vi "_USB_CAN_BI_.vi"(11 "BOARD_INFO":T1) -> (2 "change?":bool, 3 "BOARD_INFO out":T1)   [LabVIEW 2011]
panel:
  in  "new_SN":string caption="新设备序号："
  in  "ok":bool
  out "str_USB_Serial":string caption="当前设备序号："
  out "str_hw_Type":string caption="硬件类型："
  out "str_Serial_Num":string caption="板卡序列号："
  out "reserved":u8 caption="保留："
  out "can_Num":u8 caption="can通道数："
  out "irq_Num":u16 caption="保留："
  out "in_Ver":string caption="驱动库版本："
  out "dr_Ver":string caption="驱动版本："
  out "fw_Ver":string caption="软件版本："
  out "hw_Ver":string caption="硬件版本："
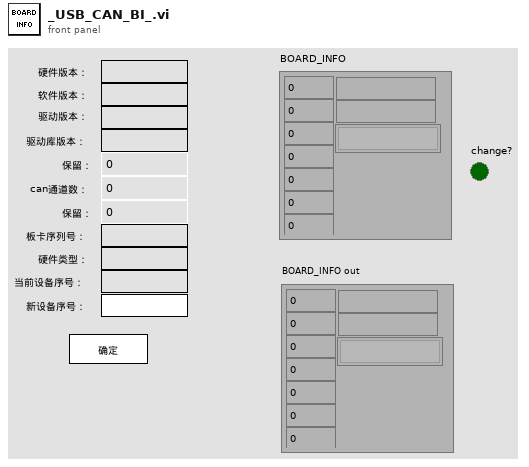
[diagram p1: front panel]
types:
  T1 = cluster{"hw_Version":u16, "fw_Version":u16, "dr_Version":u16, "in_Version":u16, "irq_Num":u16, "can_Num":u8, "reserved":u8, "str_Serial_Num":string, "str_hw_Type":string, "str_GYUsb_Serial":string[]}
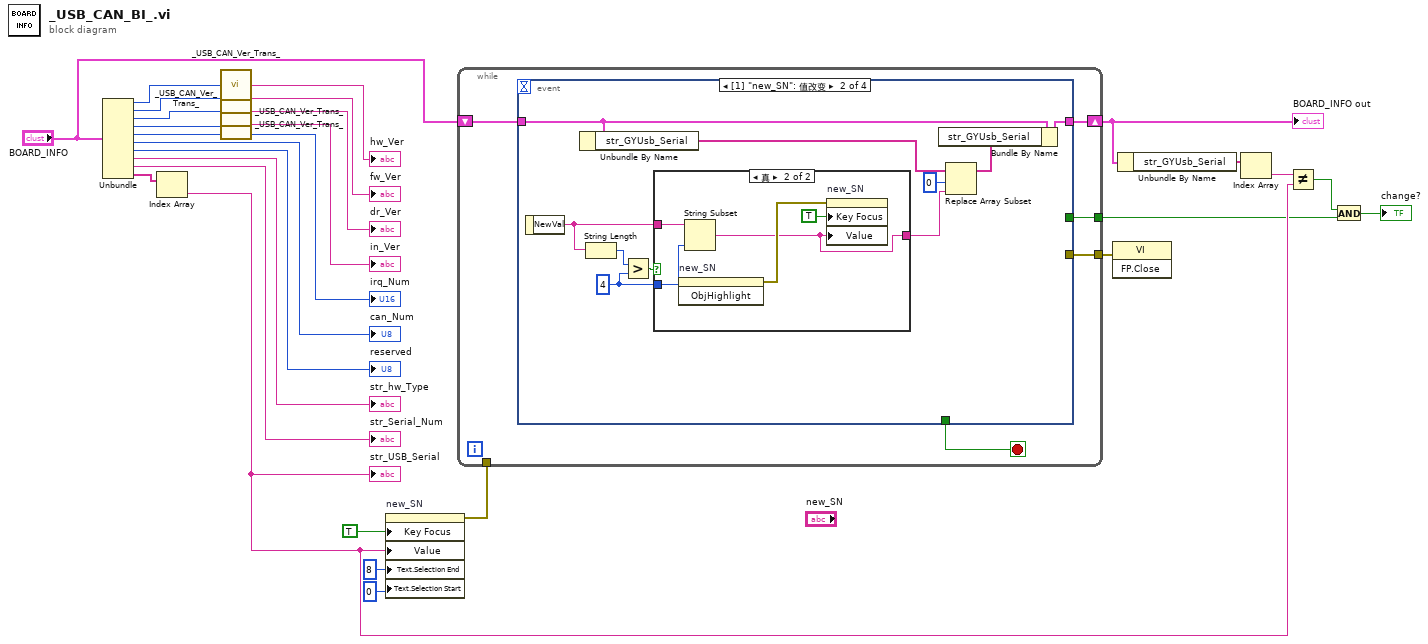
[diagram p0: block diagram]
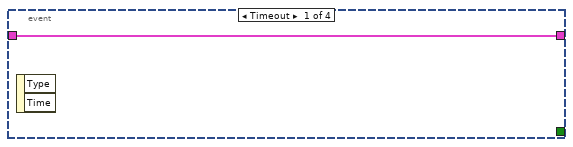
[diagram p2: hidden frame]
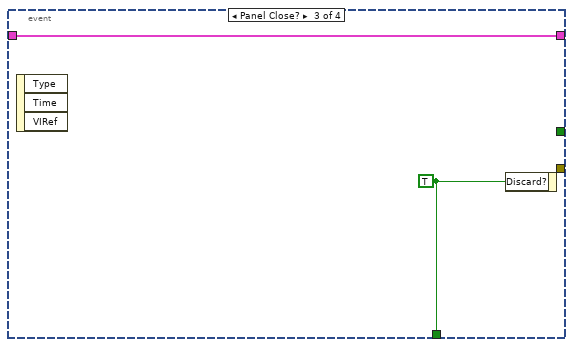
[diagram p4: hidden frame]
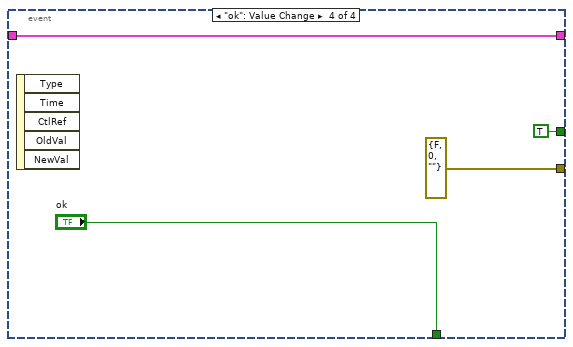
[diagram p5: hidden frame]
diagram:
  n1 = Unbundle("BOARD_INFO") -> ("hw_Version"=w20:u16, "fw_Version"=w19:u16, "dr_Version"=w18:u16, "in_Version"=w17:u16, "irq_Num"=→"irq_Num":u16, "can_Num"=→"can_Num":u8, "reserved"=→"reserved":u8, "str_Serial_Num"=→"str_hw_Type":string, "str_hw_Type"=→"str_Serial_Num":string, "str_GYUsb_Serial"=w22:string[])
  n2 = Index Array(array=w22) -> (element=w6:string)  [unwired: 1 in]
  "str_USB_Serial" <- w6
  n3 = call "_USB_CAN_Ver_Trans_.vi"("u16Ver"=w20) -> ("strVer"=→"hw_Ver":string)
  n4 = call "_USB_CAN_Ver_Trans_.vi"("u16Ver"=w19) -> ("strVer"=→"fw_Ver":string)
  n5 = call "_USB_CAN_Ver_Trans_.vi"("u16Ver"=w18) -> ("strVer"=→"dr_Ver":string)
  n6 = call "_USB_CAN_Ver_Trans_.vi"("u16Ver"=w17) -> ("strVer"=→"in_Ver":string)
  n7 = property on="new_SN" class="Str"("Key Focus"=TRUE ("键选中"), "Value"=w6, "Text.Selection End"=u32 8 ("文本.选择区域:末尾"), "Text.Selection Start"=u32 0 ("文本.选择区域:起始")) -> (error out=w11:errorcluster)  [unwired: 2 in, 1 out]
  n8 = while {
    tunnel: [w31] -> w21
    tunnel: w11 -> [_]
    shift-right: [w30] -> w9
    shift-left: "BOARD_INFO" -> [w29]
    tunnel: [w28] -> w5
    stop <- w32 stop-if-true
    n9 = event shown="[1] \"new_SN\": 值改变" {
      selector: _ -> [_ _ _ _]
      dyn-events: _ -> [_ _ _ _]
      timeout: _ -> [_ _ _ _]
      tunnel: [_ _ w51 "ok"] -> w32
      tunnel: [_ _ _ errorcluster {"status"=FALSE, "code"=0, "source"=""} ("错误输入（无错误）")] -> w31
      tunnel: [w33 w39 w50 w53] -> w30
      tunnel: w29 -> [w33 w38 w50 w53]
      tunnel: [_ _ _ TRUE ("放弃？")] -> w28
      event Timeout {
        n10 = event-data() -> ()  [unwired: 1 in, 2 out]
      }
      event "new_SN": Value Change {
        w40 = 4 ("y")
        n11 = event-data() -> ("NewVal"=w41:string)  [unwired: 1 in]
        n12 = Unbundle By Name(w38) -> ("str_GYUsb_Serial"=w37:string[])
        n13 = String Length(string=w41) -> (length=w43:i32)
        n14 = Greater?(x=w43, y=w40) -> (0:w42:bool)
        n15 = case shown="真" w42 {
          tunnel: w41 -> [w44 w49]
          tunnel: w40 -> [_ w48]
          tunnel: [w44 w45] -> w35
          frame False {
          }
          frame True {
            n16 = invoke on="new_SN" class="Str" method="ObjHighlight"() -> (error out=w46:errorcluster)  [unwired: 3 in, 2 out]
            n17 = String Subset(string=w49, length (rest)=w48) -> (substring=w45:string)  [unwired: 1 in]
            n18 = property on="new_SN" class="Str"(error in=w46, "Key Focus"=TRUE ("键选中"), "Value"=w45) -> ()  [unwired: 1 in, 2 out]
          }
        }
        n19 = Replace Array Subset(array=w37, new element=w35, index=0 ("索引")) -> (w34:string[])
        n20 = Bundle By Name(cluster=w38, "str_GYUsb_Serial"=w34) -> (w39:T1)
      }
      event Panel Close? {
        w51 = TRUE ("放弃？")
        n21 = event-data() -> ()  [unwired: 1 in, 3 out]
        n22 = event-data("Discard?"=w51) -> ()  [unwired: 1 in, 1 out]
      }
      event "ok": Value Change {
        n23 = event-data() -> ()  [unwired: 1 in, 5 out]
      }
    }
  }
  "BOARD_INFO out" <- w9
  n24 = invoke class="VI" method="FP.Close"(error in=w21) -> ()  [unwired: 2 in, 3 out]
  n25 = Unbundle By Name(w9) -> ("str_GYUsb_Serial"=w8:string[])
  n26 = Index Array(array=w8) -> (element=w7:string)  [unwired: 1 in]
  n27 = Not Equal?(x=w7, y=w6) -> (x != y?=w4:bool)
  n28 = And(x=w4, y=w5) -> (x .and. y?=→"change?":bool)
